vi "niTuner Close.vi"(8 "error in":errorcluster, 11 "taskID in":i32=1 format="%.0x") -> (0 "error out":errorcluster {"code" format="%.0x"})   [LabVIEW 2011]
doc: "This VI closes the instrument I/O session."
uses:
  nipxi5600u.dll
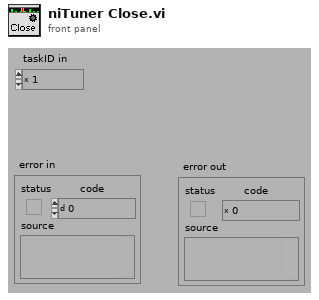
[diagram p1: front panel]
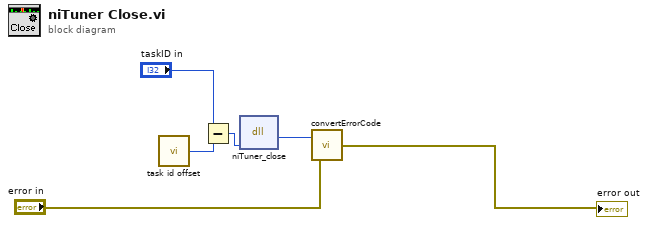
[diagram p0: block diagram]
diagram:
  n1 = call <instrlib>:"task id offset.vi"() -> ("taskID offset"=w1:i32)
  n2 = Subtract(x="taskID in", y=w1) -> (x-y=w2:i32)
  n3 = dll-call lib="nipxi5600u.dll" fn="niTuner_close"("taskID"=w2) -> (w3:i32)  [unwired: 4 in, 2 out]
  n4 = call <instrlib>:"convertErrorCode.vi"("error in"="error in", "error code"=w3) -> ("error out"=→"error out":errorcluster)
